vi "Process Image for Target GrayScale.vi"(0 "Src Image":T2, 1 "Color Mode":u16(ring)=2 items=["RGB", "HSL", "HSV", "HSI"], 7 "Range":cluster{"Lower value":sgl, "Upper value":sgl}={"Lower value"=150.0, "Upper value"=255.0} {"Lower value" scale=0.0..255.0; "Upper value" scale=0.0..255.0}, 11 "Area Cutoff %":dbl=0.05) -> (4 "Src Image Out":T2, 8 "Threshold":T2, 15 "Particles":T1(array[cluster]))   [LabVIEW 2013]
doc: "Use color, rectangularity, and aspect ratio to identify and describe potential strips of retroreflective material within the image."
uses:
  <vilib>/vision/Image Controls.llb/IMAQ Image.ctl
  <vilib>/vision/NI_Vision_Development_Module.lvlib
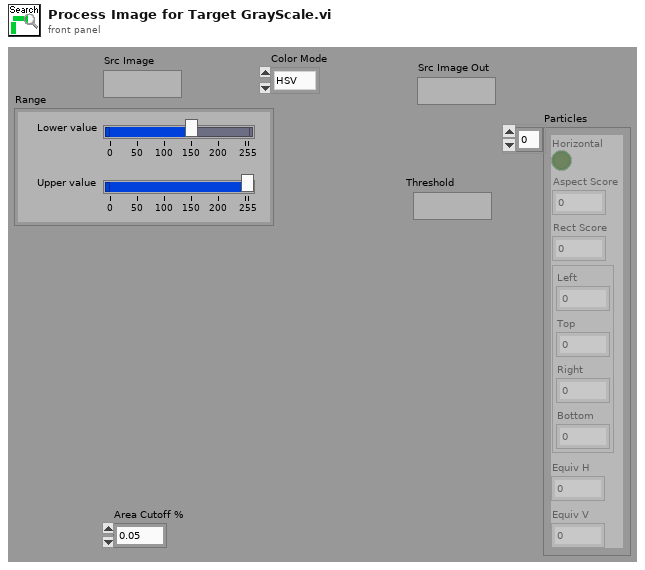
[diagram p1: front panel]
types:
  T1 = cluster{"Horizontal":bool, "Aspect Score":dbl, "Rect Score":dbl, cluster{"Left":dbl, "Top":dbl, "Right":dbl, "Bottom":dbl}, "Equiv H":dbl, "Equiv V":dbl}[]
  T2 = typedef "IMAQ Image.ctl" = refnum<image>
  T3 = typedef "Image Type" = u32
  T4 = typedef "Particle Parameters" = i32
  T5 = cluster{"Numeric":dbl, "Numeric":dbl, "Numeric":dbl, "Numeric":dbl}
  T6 = cluster{"Horizontal":bool, "Score":dbl, "Score":dbl, cluster{"Numeric":dbl, "Numeric":dbl, "Numeric":dbl, "Numeric":dbl}, "Numeric":dbl, "Numeric":dbl}
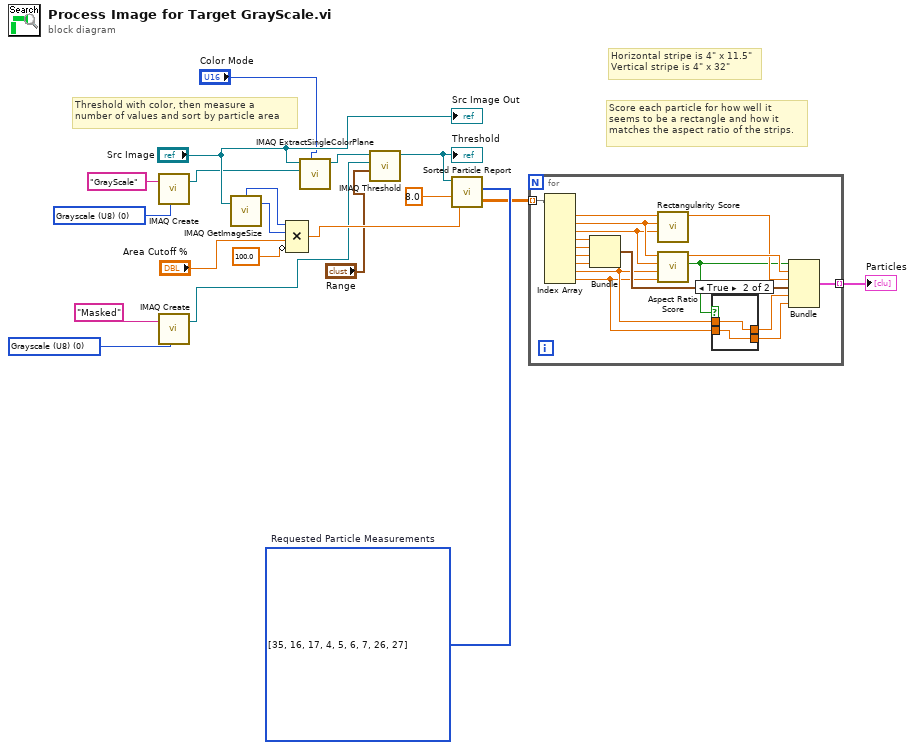
[diagram p0: block diagram]
diagram:
  w4 = T3 0 items=["Grayscale (U8)", "Grayscale (I16)", "Grayscale (SGL)", "Complex (CSG)", "RGB (U32)", "HSL (U32)", "RGB (U64)", "Grayscale (U16)"] ("Image Type")
  w12 = T4[] [35, 16, 17, 4, 5, 6, 7, 26, 27] items=["Center of Mass X", "Center of Mass Y", "First Pixel X", "First Pixel Y", "Bounding Rect Left", "Bounding Rect Top", "Bounding Rect Right", "Bounding Rect Bottom", "Max Feret Diameter Start X", "Max Feret Diameter Start Y", "Max Feret Diameter End X", "Max Feret Diameter End Y", "Max Horiz. Segment Length Left", "Max Horiz. Segment Length Right", "Max Horiz. Segment Length Row", "-", "Bounding Rect Width", "Bounding Rect Height", "Bounding Rect Diagonal", "Perimeter", "Convex Hull Perimeter", "Holes' Perimeter", "Max Feret Diameter", "Equivalent Ellipse Major Axis", "Equivalent Ellipse Minor Axis", "Equivalent Ellipse Minor Axis (Feret)", "Equivalent Rect Long Side", "Equivalent Rect Short Side", "Equivalent Rect Diagonal", "Equivalent Rect Short Side (Feret)", "Average Horiz. Segment Length", "Average Vert. Segment Length", "Hydraulic Radius", "Waddel Disk Diameter", "-", "Area", "Holes' Area", "Particle & Holes' Area", "Convex Hull Area", "Image Area", "-", "Number of Holes", "Number of Horiz. Segments", "Number of Vert. Segments", "-", "Orientation", "Max Feret Diameter Orientation", "-", "% Area/Image Area", "% Area/(Particle & Holes' Area)", "Ratio of Equivalent Ellipse Axes", "Ratio of Equivalent Rect Sides", "-", "Elongation Factor", "Compactness Factor", "Heywood Circularity Factor", "Type Factor", "-", "Sum X", "Sum Y", "Sum XX", "Sum XY", "Sum YY", "Sum XXX", "Sum XXY", "Sum XYY", "Sum YYY", "-", "Moment of Inertia XX", "Moment of Inertia XY", "Moment of Inertia YY", "Moment of Inertia XXX", "Moment of Inertia XXY", "Moment of Inertia XYY", "Moment of Inertia YYY", "Norm. Moment of Inertia XX", "Norm. Moment of Inertia XY", "Norm. Moment of Inertia YY", "Norm. Moment of Inertia XXX", "Norm. Moment of Inertia XXY", "Norm. Moment of Inertia XYY", "Norm. Moment of Inertia YYY", "Hu Moment 1", "Hu Moment 2", "Hu Moment 3", "Hu Moment 4", "Hu Moment 5", "Hu Moment 6", "Hu Moment 7"]  # Requested Particle Measurements
  w19 = T3 0 items=["Grayscale (U8)", "Grayscale (I16)", "Grayscale (SGL)", "Complex (CSG)", "RGB (U32)", "HSL (U32)", "RGB (U64)", "Grayscale (U16)"] ("Image Type")
  # "Score each particle for how well it\nseems to be a rectangle and how it\nmatches the aspect ratio of the strips."
  # "Horizontal stripe is 4\" x 11.5\"\nVertical stripe is 4\" x 32\""
  # "Threshold with color, then measure a\nnumber of values and sort by particle area"
  n1 = call "IMAQ Create"("Image Name"="GrayScale", "Image Type"=w19) -> ("New Image"=w8:T2)  [unwired: 3 in, 1 out]
  n2 = call "IMAQ Create"("Image Name"="Masked", "Image Type"=w4) -> ("New Image"=w2:T2)  [unwired: 3 in, 1 out]
  n3 = call "IMAQ GetImageSize"("Image"="Src Image") -> ("Y Resolution"=w15:i32, "X Resolution"=w16:i32)  [unwired: 3 in, 1 out]
  n4 = Compound Arithmetic op=MULTIPLY(w16, w15, "Area Cutoff %", invert 100.0 ("value")) -> (w13:dbl)
  n5 = call "IMAQ ExtractSingleColorPlane"("Color Plane"="Color Mode", "Image Dst"=w8, "Image Src"="Src Image") -> ("Image Dst Out"=w6:T2)  [unwired: 1 in, 7 out]
  n6 = call "IMAQ Threshold"("Range"="Range", "Image Dst"=w2, "Image Src"=w6) -> ("Image Dst Out"=w1:T2)  [unwired: 3 in, 5 out]
  "Threshold" <- w1
  n7 = call "Sorted Particle Report.vi"("Area Size Limit"=w13, "Particle Count Limit"=8.0, "Pixel Measurements"=w12, "Image in"=w1) -> ("Sorted Data"=w11:dbl[][])  [unwired: 1 out]
  n8 = for {
    tunnel: w11 -> [w37] mode=indexing
    tunnel: [w27] -> w10 mode=indexing
    n9 = Index Array(array=w37) -> (element #1=w36:dbl, element #2=w31:dbl, element #3=w30:dbl, element #4=w35:dbl, element #5=w34:dbl, element #6=w33:dbl, element #7=w32:dbl, element #8=w22:dbl, element #9=w21:dbl)  [unwired: 9 in]
    n10 = Bundle("Numeric"=w35, "Numeric"=w34, "Numeric"=w33, "Numeric"=w32) -> (w26:T5)  [unwired: 1 out]
    n11 = call "Rectangularity Score.vi"("Height"=w30, "Width"=w31, "Area"=w36) -> ("Score"=w28:dbl)  [unwired: 8 in]
    n12 = call "Aspect Ratio Score.vi"("Equivalent Rect Short"=w21, "Equivalent Rect Long"=w22, "Height"=w30, "Width"=w31) -> ("Horizontal"=w23:bool, "Score"=w29:dbl)  [unwired: 6 in]
    n13 = case shown="True" w23 {
      tunnel: w21 -> [w38 w41]
      tunnel: w22 -> [w39 w40]
      tunnel: [w39 w41] -> w25
      tunnel: [w38 w40] -> w24
      frame False {
      }
      frame True {
      }
    }
    n14 = Bundle("Horizontal"=w23, "Score"=w29, "Score"=w28, w26, "Numeric"=w24, "Numeric"=w25) -> (w27:T6)  [unwired: 1 out]
  }
  "Particles" <- w10
  "Src Image Out" <- "Src Image"
